vi "read.raw.file.vi"(10 "Raw File":string, 11 "Path":path) -> (3 "data":u8[](array[numeric]))   [LabVIEW 2020]
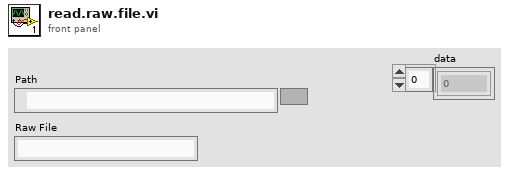
[diagram p1: front panel]
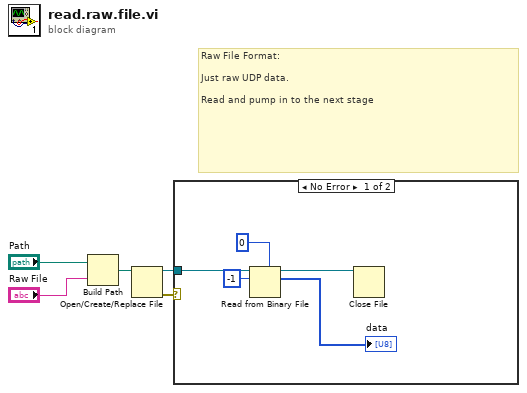
[diagram p0: block diagram]
diagram:
  # "Raw File Format:\n\nJust raw UDP data.\n\nRead and pump in to the next stage"
  n1 = Build Path(base path="Path", name or relative path="Raw File") -> (appended path=w3:path)
  n2 = Open/Create/Replace File(file path (use dialog)=w3) -> (refnum out=w1:refnum<file>, error out=w2:errorcluster)  [unwired: 5 in, 1 out]
  n3 = case shown="No Error" w2 {
    tunnel: w1 -> [w10 _]
    frame No Error {
      n4 = Read from Binary File(5:u8 0 ("count (1)"), 10:-1 ("count (1)"), 11:w10) -> (2:→"data":u8[], 3:w7:refnum<file>)  [unwired: 3 in, 2 out]
      n5 = Close File(refnum=w7) -> ()  [unwired: 1 in, 2 out]
    }
    frame Error {
    }
  }
